vi "Set_Undefined_Destination_Post_Linker.vi"(6 "linkerInfo":T2, 7 "computed dests":i32[](array[numeric]), 8 "error in (no error)":errorcluster, 9 "Linker:Read Info From File":T3(array[cluster]), 10 "destination in":i32, 11 "AB_Source_PackedItem in":refnum<class "AB_Source_PackedItem.lvclass">) -> (0 "error out":errorcluster, 2 "destination out":i32, 3 "AB_Source_PackedItem out":refnum<class "AB_Source_PackedItem.lvclass">)   [LabVIEW 2020, in "AB_Source_PackedItem.lvclass"]
uses:
  <vilib>/AppBuilder/AB_Classes/Source/PackedItem/AB_Source_PackedItem.lvclass
  <vilib>/Utility/lvfile.llb/LVFileType.ctl
  <vilib>/Utility/lvfile.llb/NI_FileType.lvlib
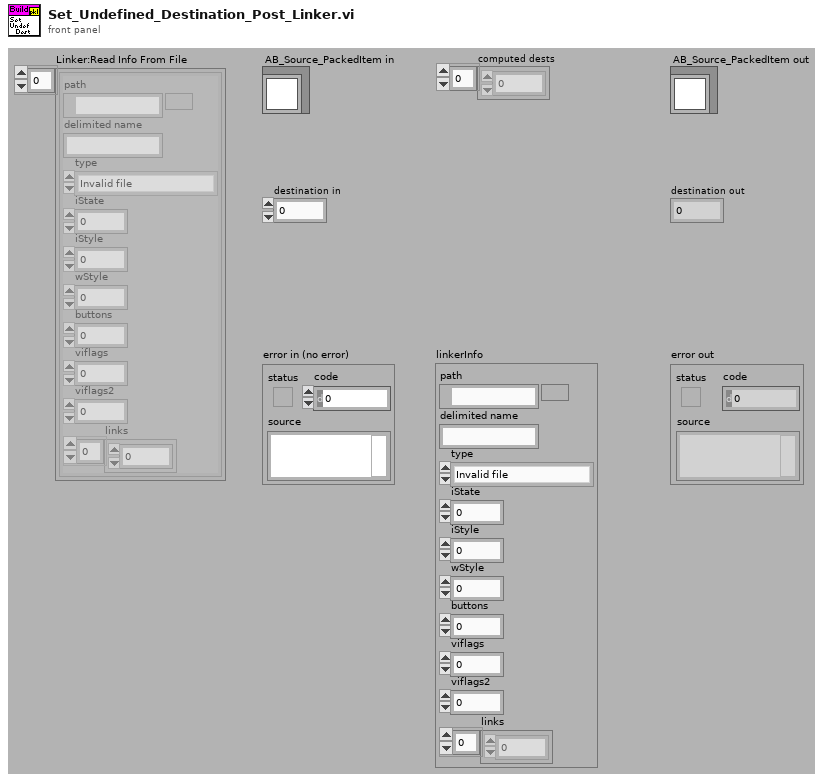
[diagram p1: front panel]
types:
  T1 = typedef "NI_FileType.lvlib/LVFileType.ctl" = enum32{"Invalid file", "Unknown type", "Instrument", "Control", "Polymorphic VI", "Project", "Library", "LVClass", "XControl", "XNode", "Shared library", ".NET assembly", "ActiveX interface", "CIN", "Run-time menu", "Palette menu", "Help file", "LLB", "XNode Edit Dependency", "Class Private Data Control", "Statechart", "MathScript .m file", "Ladder Diagram", "LVLibp", "XNode Build Dependency"}
  T2 = cluster{"path":path, "delimited name":string, "type":T1, "iState":u32, "iStyle":u16, "wStyle":u16, "buttons":u16, "viflags":u32, "viflags2":u32, "links":u32[]}
  T3 = cluster{"path":path, "delimited name":string, "type":T1, "iState":u32, "iStyle":u16, "wStyle":u16, "buttons":u16, "viflags":u32, "viflags2":u32, "links":u32[]}[]
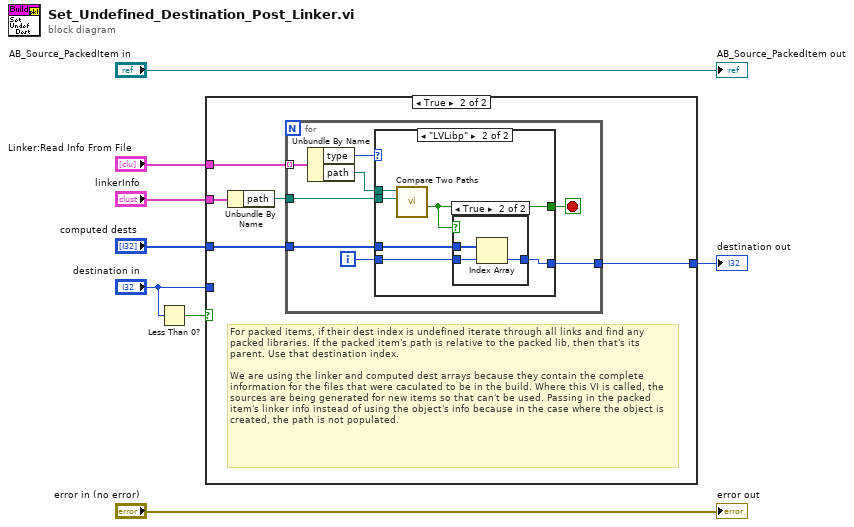
[diagram p0: block diagram]
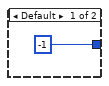
[diagram p3: hidden frame]
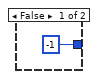
[diagram p4: hidden frame]
diagram:
  n1 = Less Than 0?(x="destination in") -> (x < 0?=w4:bool)
  n2 = case shown="True" w4 {
    tunnel: [w9 w14] -> w7
    tunnel: "destination in" -> [w9 _]
    tunnel: "Linker:Read Info From File" -> [_ w13]
    tunnel: "linkerInfo" -> [_ w12]
    tunnel: "computed dests" -> [_ w10]
    frame False {
    }
    frame True {
      # "For packed items, if their dest index is undefined iterate through all links and find any packed libraries. If the packed item's path is relative to the packed lib, then that's its parent. Use that destination index. \n\nWe are using the linker and computed dest arrays because they contain the complete information for the files that were caculated to be in the build. Where this VI is called, the sources are being generated for new items so that can't be used. Passing in the packed item's linker info instead of using the object's info because in the case where the object is created, the path is not populated."
      n3 = Unbundle By Name(w12) -> ("path"=w11:path)
      n4 = for {
        tunnel: w11 -> [w22]
        tunnel: [w20] -> w14
        tunnel: w13 -> [w19] mode=indexing
        tunnel: w10 -> [w16]
        i -> [w15]
        stop <- w21 stop-if-true
        n5 = Unbundle By Name(w19) -> ("type"=w18:T1, "path"=w17:path)
        n6 = case shown="\"LVLibp\"" w18 {
          tunnel: w17 -> [_ w29]
          tunnel: w22 -> [_ w28]
          tunnel: [_ w27] -> w21
          tunnel: [-1 ("destinationIndex") w24] -> w20
          tunnel: w16 -> [_ w26]
          tunnel: w15 -> [_ w25]
          frame Default {
          }
          frame "LVLibp" {
            n7 = call <vilib>:"Compare Two Paths.vi"("Path 2"=w28, "Path 1"=w29) -> ("Path 2 Relative to Path 1?"=w27:bool)  [unwired: 6 in, 3 out]
            n8 = case shown="True" w27 {
              tunnel: w26 -> [_ w33]
              tunnel: w25 -> [_ w32]
              tunnel: [-1 w31] -> w24
              frame False {
              }
              frame True {
                n9 = Index Array(array=w33, index=w32) -> (element=w31:i32)
              }
            }
          }
        }
      }
    }
  }
  "destination out" <- w7
  "error out" <- "error in (no error)"
  "AB_Source_PackedItem out" <- "AB_Source_PackedItem in"
